vi "String display_0.vi"() -> ()   [LabVIEW 2015]
panel:
  in  "Tab Control":enum32{"Page 1", "Page 2"}(tab)
  in  "String":string="hwbhwdbcwkj\nwwecercerc\neer\nc\nerevvrtg3rwvrt\nv42\nrf24rf424"
  out "concatenated string":string
  # "String display"
  # "Pardeep Kumar"
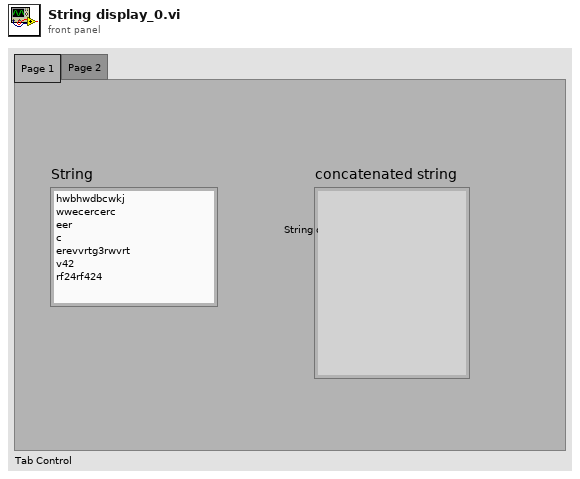
[diagram p1: front panel]
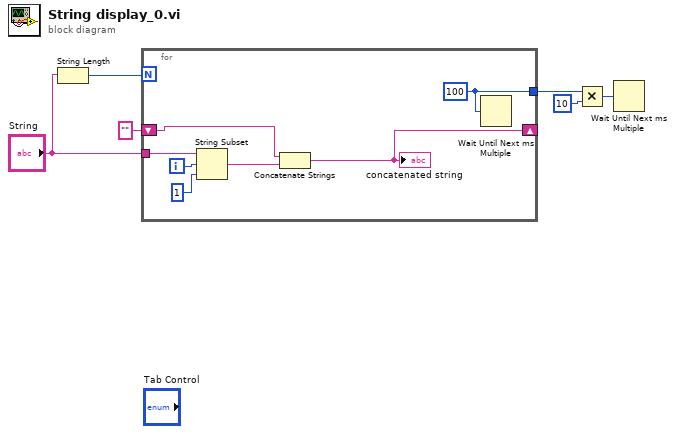
[diagram p0: block diagram]
diagram:
  n1 = String Length(string="String") -> (length=w6:i32)
  n2 = for {
    N: w6 -> [_]
    tunnel: "String" -> [w13]
    shift-right: [w9] -> _
    shift-left: "" -> [w8]
    tunnel: [w7] -> w5
    i -> [w12]
    w7 = u32 100 ("millisecond multiple")
    n3 = String Subset(string=w13, offset (0)=w12, length (rest)=1 ("length (rest)")) -> (substring=w10:string)
    n4 = Concatenate Strings "Concatenate Strings"(w8, w10) -> (w9:string)
    "concatenated string" <- w9
    n5 = Wait Until Next ms Multiple(millisecond multiple=w7) -> ()  [unwired: 1 out]
  }
  n6 = Multiply(x=w5, y=u32 10) -> (x*y=w3:u32)
  n7 = Wait Until Next ms Multiple(millisecond multiple=w3) -> ()  [unwired: 1 out]
